vi "Module Identities.vi"(8 "error in (no error)":errorcluster, 11 "Event Viewer Module in":refnum<class "Event Viewer Module.lvclass">) -> (0 "error out":errorcluster, 2 "Identities":refnum<class "Identity.lvclass">[](array[class]), 3 "Event Viewer Module out":refnum<class "Event Viewer Module.lvclass">)   [LabVIEW 2020, in "VolatusGUI.lvlib" / "Event Viewer Module.lvclass"]
uses:
  Event Viewer Module.lvclass
  Volatus/Identity/Identity.lvclass
  Event Viewer Identity/Event Viewer Identity.lvclass
  C:/dev/lv20CE/relink/lv-volatus/Volatus/Identity/Identity.lvclass
  Event Viewer Module.lvclass/Event Viewer Module.ctl
  C:/dev/lv20CE/relink/lv-volatus/VolatusGUI/Event Viewer Identity/Event Viewer Identity.lvclass
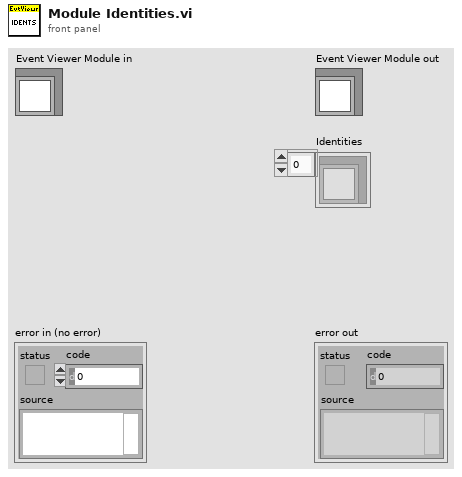
[diagram p1: front panel]
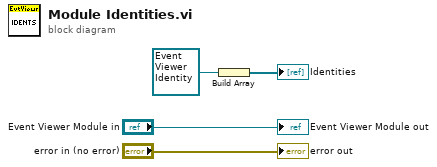
[diagram p0: block diagram]
diagram:
  n1 = Build Array(refnum<class "Event Viewer Identity.lvclass"> refnum ("VolatusGUI:Event Viewer Identity.lvclass")) -> (→"Identities":refnum<class "Event Viewer Identity.lvclass">[])
  "error out" <- "error in (no error)"
  "Event Viewer Module out" <- "Event Viewer Module in"
